vi "acquireValue.vi"(8 "error in (no error)":errorcluster, 10 "nextSample?":bool, 11 "rejectedCommand in":refnum<class "rejectedCommand.lvclass">) -> (0 "error out":errorcluster, 1 "function return":i32, 2 "variantData":variant, 3 "rejectedCommand out":refnum<class "rejectedCommand.lvclass">)   [LabVIEW 2016, in "SALLV_EXA_Messaging.lvlib" / "rejectedCommand.lvclass"]
uses:
  rejectedCommand.lvclass
  rejectedCommand.lvclass/rejectedCommand.ctl
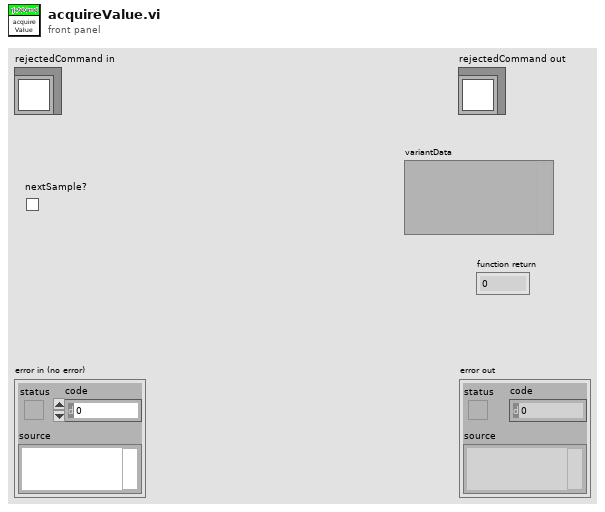
[diagram p1: front panel]
types:
  T1 = typedef "SALLV_EXA.lvlib/logevent_rejectedCommand.ctl" = cluster{"command":string, "state":string, "timestamp":dbl, "priority":i32}
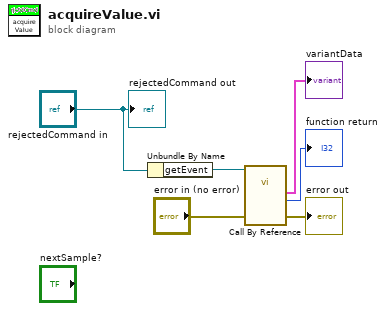
[diagram p0: block diagram]
diagram:
  n1 = Unbundle By Name("rejectedCommand in") -> ("getEvent"=w6:refnum<vi>)
  n2 = call-by-ref "?"(reference=w6, "error in (no error)"="error in (no error)") -> ("error out"=→"error out":errorcluster, "function return"=→"function return":i32, "logevent_rejectedCommand_Ctl out"=→"variantData":T1)  [unwired: 9 in, 2 out]
  "rejectedCommand out" <- "rejectedCommand in"
